vi "RT Driver VI.vi"(7 "Operation":T1, 11 "Device Reference in":T2 format="%.0x") -> (0 "Error Code":i32)   [LabVIEW 2019, in "Protection and Counter Addon Engine.lvlib"]
uses:
  Protection and Counter Addon Engine.lvlib
  <vilib>/NI VeriStand/Custom Device API/Custom Device Item Ref.ctl
  <vilib>/NI VeriStand/Custom Device API/Hardware Interface Driver VI Operation.ctl
  <vilib>/NI/NIVS Inline Async API/_VS Inline Async API/VS Inline Async API/VS Inline Async API.lvclass
  Types/RT Async Engine Settings.ctl
  SubModules/Frame-Protection-Support/Source/Engine/Types/RT Frame Settings.ctl
  SubModules/Frame-Protection-Support/Source/Shared/Types/Exported Frame Type.ctl
  SubModules/Frame-Protection-Support/Source/Engine/Types/RT Protection Configuration.ctl
  SubModules/Frame-Protection-Support/Source/Shared/Types/Protection Type.ctl
  SubModules/Frame-Protection-Support/Source/Shared/Types/XNET Signal Configuration.ctl
  SubModules/Frame-Protection-Support/Source/Shared/Types/Exported Counter Settings.ctl
  SubModules/Frame-Protection-Support/Source/Shared/Types/Exported Event Trigger Type.ctl
  Addon Shared/Types/XNET Settings.ctl
  SubModules/Frame-Protection-Support/Source/Shared/Types/RT_Incoming_Signal_Info.ctl
  SubModules/Frame-Protection-Support/Source/Shared/Types/RT Exported Signal Settings.ctl
  Addon Shared/Types/Exported.OnCompile.ctl
  SubModules/Frame-Protection-Support/Source/Shared/Types/Exported Frame Settings.ctl
  SubModules/Frame-Protection-Support/Source/Shared/Types/Exported Protection Settings.ctl
  Addon Shared/Types/986x.ctl
  SubModules/Frame-Protection-Support/Source/Shared/Types/Incoming Signal Info.ctl
  SubModules/Frame-Protection-Support/Source/Shared/Types/Exported Signal Settings.ctl
  <vilib>/NI/NIVS Inline Async API/_VS Inline Async API/VS Inline Async API/Types/Error Handling Settings.ctl
  <vilib>/NI/NIVS Inline Async API/_VS Inline Async API/VS Inline Async API/VS Inline Async API.lvclass/VS Inline Async API.ctl
  <vilib>/NI/NIVS Inline Async API/_Data Access Engine/Data Access Engine/Data Access Engine.lvclass/Data Access Engine.ctl
  <vilib>/NI/NIVS Inline Async API/_Data Access Engine/Access Type Classes/Write/Write.lvclass/Write.ctl
  <vilib>/NI/NIVS Inline Async API/_Data Access Engine/Access Type Classes/ReadWrite/ReadWrite.lvclass/ReadWrite.ctl
  <vilib>/NI/NIVS Inline Async API/_Data Access Engine/Access Type Classes/Read/Read.lvclass/Read.ctl
  <vilib>/NI/NIVS Inline Async API/_Data Access Engine/Data Access Engine/Methods/Data.Engine.Read Data from HW.vi
  <vilib>/NI/NIVS Inline Async API/_VS Inline Async API/Error Handling Process/SubVIs/Error.GetError.vi
  <vilib>/NI/NIVS Inline Async API/_Data Access Engine/Data Access Engine/Methods/Data.Engine.Write Data to HW.vi
  <vilib>/NI/NIVS Inline Async API/_Data Access Engine/Access Type Classes/ReadWrite/ReadWrite.EngineData.vi
  <vilib>/NI/NIVS Inline Async API/_Data Access Engine/Access Type Classes/Write/Write.EngineData.vi
  <vilib>/NI/NIVS Inline Async API/_Data Access Engine/Access Type Classes/Read/Read.EngineData.vi
  <vilib>/NI VeriStand/Custom Device API/NI VeriStand - Get Channel Value by Data Reference.vi
  <vilib>/NI VeriStand/Custom Device API/NI VeriStand - Set Channel Value by Data Reference.vi
  <vilib>/NI VeriStand/Custom Device API/NI VeriStand - Get Channel Values by Block Data Reference.vi
  Addon Shared/SubVIs/GUID Lookup.vi
  <vilib>/NI VeriStand/Custom Device API/Get Item Property (Variant).vi
  <vilib>/Utility/SystemLogging/Write to System Log.vi
  <vilib>/NI VeriStand/Custom Device API/Global Data Refs.vi
  <vilib>/NI VeriStand/Custom Device API/Custom Device API.lvlib
  Addon Shared/Protection and Counter Addon Shared.lvlib
  SubModules/Frame-Protection-Support/Source/Shared/Protection and Counter Support Shared.lvlib
  <vilib>/NI VeriStand/Custom Device Tools/Custom Device Utility Library/Custom Device Utility Library.lvlib
  SubModules/Frame-Protection-Support/Source/Engine/Protection and Counter Support Engine.lvlib
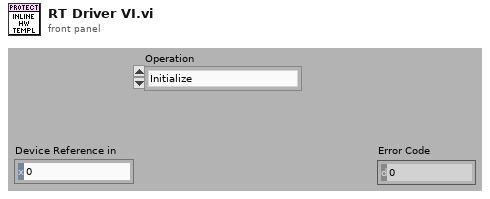
[diagram p1: front panel]
types:
  T1 = typedef "Custom Device API.lvlib/Hardware Interface Driver VI Operation.ctl" = enum16{"Initialize", "Start", "Read Data from HW", "Write Data to HW", "Close"}
  T2 = typedef "Custom Device API.lvlib/Custom Device Item Ref.ctl" = u64
  T3 = typedef "Protection and Counter Addon Engine.lvlib/RT Async Engine Settings.ctl" = cluster{"Name":string, "Priority":i32, "CAN Session":refnum<k21>, "Frame Count":i32, "Frames":T4[], "FPGA Session":u32, "XNET Settings":T11, "Incoming Frame Session":refnum<k21>, "Incoming Session Invalid":bool, "Incoming Signal Info":T12, "Signal Values":dbl[]}
  T4 = typedef "Protection and Counter Support Engine.lvlib/RT Frame Settings.ctl" = cluster{"Type":T5, "Frame ID":u32, "Payload Length":u32, "VS Offset":i32, "VS Length":i32, "Frame Conversion":refnum<k21>, "Frame.Data":dbl[], "Generation Period":u32, "Time Since Last Generation":u32, "Generation Iterations":u32, "Generation Counter":u32, "Has Protection?":bool, "Protection Configurations":T6[], "Has Counter?":bool, "Counter Configurations":T9[], "Has Disable?":bool, "Disable VS Index":i32, "Transmit Trigger":T10, "Trigger VS Index":i32}
  T5 = typedef "Protection and Counter Support Shared.lvlib/Exported Frame Type.ctl" = enum16{"Periodic", "Event", "Periodic/Event"}
  T6 = typedef "Protection and Counter Support Engine.lvlib/RT Protection Configuration.ctl" = cluster{"Protection Frame Index":i32, "Protection Type":T7, "Data Indeces":i32[], "Data Array":dbl[], "Check Sum Conversion":refnum<k21>, "CRC Channels":T8[], "Protection VS Index":i32, "Counter Data Index":i32, "Override Index":i32, "Override Value Index":i32}
  T7 = typedef "Protection and Counter Support Shared.lvlib/Protection Type.ctl" = enum16{"Arb ID + Bytes Checksum with Inversion", "Arb ID + Bytes CRC with Inversion", "Reversed Raw Signal Checksum with Inversion", "Concatenated Two's Compliment"}
  T8 = typedef "Protection and Counter Support Shared.lvlib/XNET Signal Configuration.ctl" = cluster{"Start Bit":i32, "Name":string, "Number of bits":i32, "Scale":dbl, "Offset":dbl, "Data Type":u32, "Counter":bool}
  T9 = typedef "Protection and Counter Support Shared.lvlib/Exported Counter Settings.ctl" = cluster{"Frame Index":i32, "Max Count":dbl, "VS Index":i32, "Bit Length":i64, "Override Index":i32, "Override Value Index":i32}
  T10 = typedef "Protection and Counter Support Shared.lvlib/Exported Event Trigger Type.ctl" = enum16{"Channel value change", "Trigger channel (not zero)", "Channel value change or trigger channel (not zero)", "Trigger channel (any value change)", "Channel value change or trigger channel (any value change)"}
  T11 = typedef "Protection and Counter Addon Shared.lvlib/XNET Settings.ctl" = cluster{"Database":refnum<k21>, "Cluster":refnum<k21>, "Port":string, "Baud rate [Bd]":u64, "Termination":u32, "CAN I/O Mode":u32, "FD Baud rate [Bd]":u64, "Priority":i32, "Use Legacy":bool, "FD ISO Mode":u32}
  T12 = typedef "RT_Incoming_Signal_Info.ctl" = cluster{"Signal_Valid_Values":dbl[], "Signal Names":string[], "Signal Settings Out":T13[], "Frame Receive Time Values":timestamp[], "ProtCtr Sig Values":dbl[], "All Sig Values":dbl[]}
  T13 = typedef "RT Exported Signal Settings.ctl" = cluster{"Is Protection":bool, "Is Counter":bool, "Signal Name":string, "Counter Configuration":T9, "Valid_Sig_Ref_Index":i32, "Frame ID":u32, "Payload Length":u32, "Protection Configuration":T6, "Frame Index":i32, "All Signal Index":i32}
  T14 = cluster{"Process":refnum<class "VS Inline Async API.lvclass">, "RT Configuration":T3}
  T15 = typedef "VS Inline Async API.lvlib/VS Inline Async API.lvclass/Error Handling Settings.ctl" = cluster{"Write to SystemLog (F)":bool}
  T16 = typedef "Protection and Counter Addon Shared.lvlib/Exported.OnCompile.ctl" = cluster{"Name":string, "XNET Settings":T11, "Frames":T17[], "986x Support":T19, "Incoming Signal Info":T20, "Incoming Frames":T17[]}
  T17 = typedef "Protection and Counter Support Shared.lvlib/Exported Frame Settings.ctl" = cluster{"Type":T5, "Frame ID":u32, "Payload Length":u32, "Signal XNET Paths":string[], "Frame.PrevData":dbl[], "VS Offset":i32, "VS Length":i32, "Generation Period":u32, "Has Protection?":bool, "Protection Configurations":T18[], "Has Counter":bool, "Counter Configurations":T9[], "Has Disable?":bool, "Disable VS Index":i32, "Transmit Trigger":T10, "Trigger VS Index":i32}
  T18 = typedef "Protection and Counter Support Shared.lvlib/Exported Protection Settings.ctl" = cluster{"Protection Frame Index":i32, "Protection Type":T7, "Data Indeces":i32[], "Initialized Data Array":dbl[], "Protection Signal XNET Paths":string[], "CRC Channels":T8[], "Protection VS Update Index":i32, "Override Index":i32, "Override Value Index":i32}
  T19 = typedef "Protection and Counter Addon Shared.lvlib/986x.ctl" = cluster{"Enable":bool, "RIO Device":string, "Bitfile":path}
  T20 = typedef "Incoming Signal Info.ctl" = cluster{"Signal Settings Out":T21[], "Signal_Valid_Values":dbl[], "Signal Names":string[], "ProtCtrValues":dbl[], "AllSigValues":dbl[]}
  T21 = typedef "Exported Signal Settings.ctl" = cluster{"Is Protection":bool, "Is Counter":bool, "Signal Name":string, "Counter Configuration":T9, "Protection Configuration":T18, "Valid_Sig_Ref_Index":i32, "Frame ID":u32, "Payload Length":u32, "Frame Index":i32, "All Signal Index":i32}
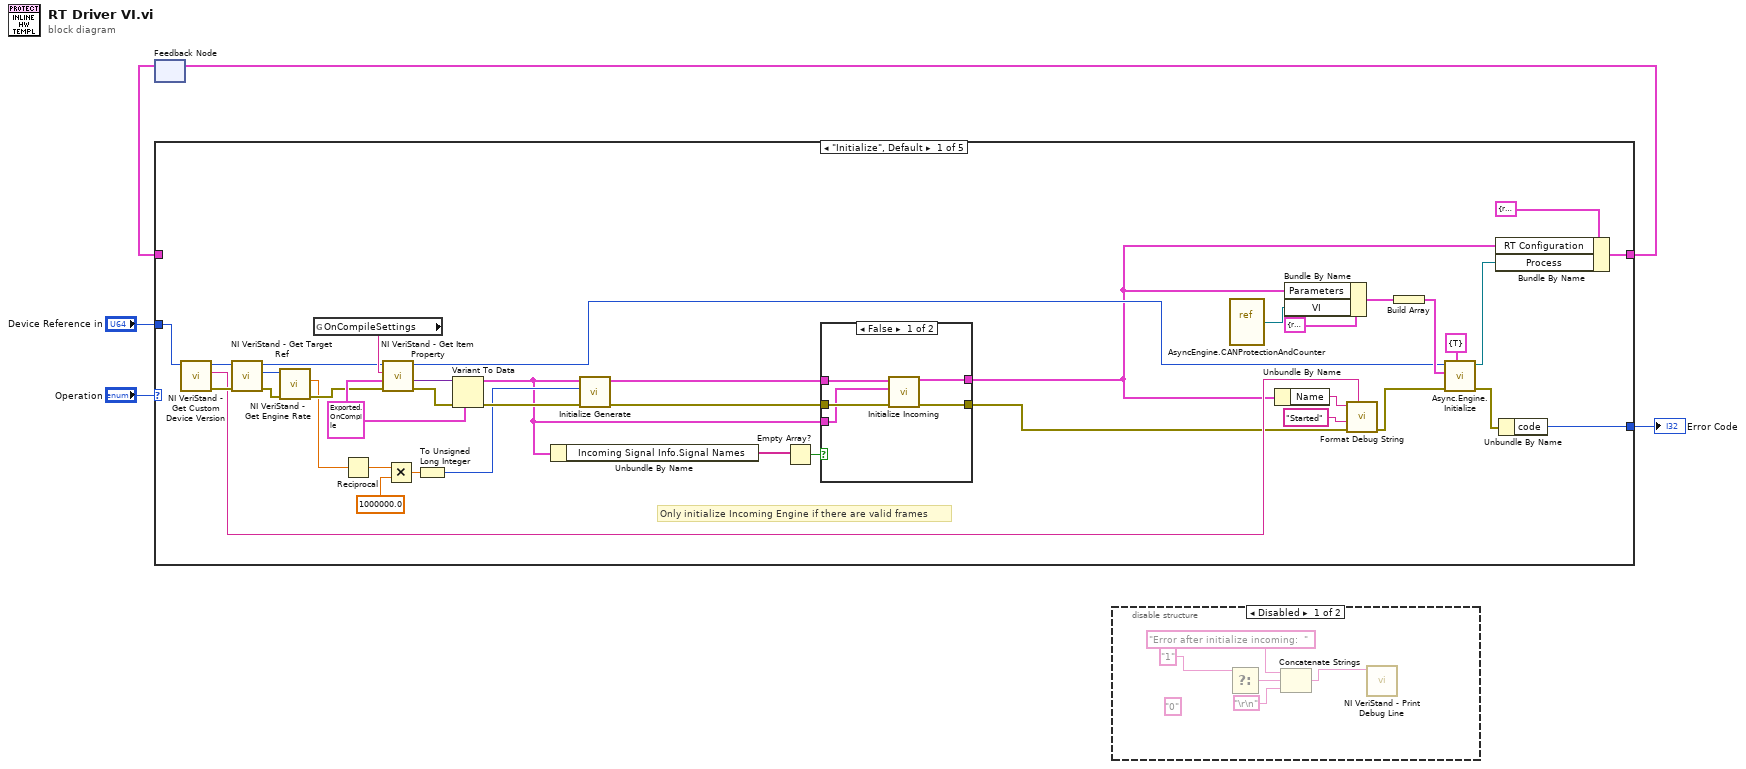
[diagram p0: block diagram]
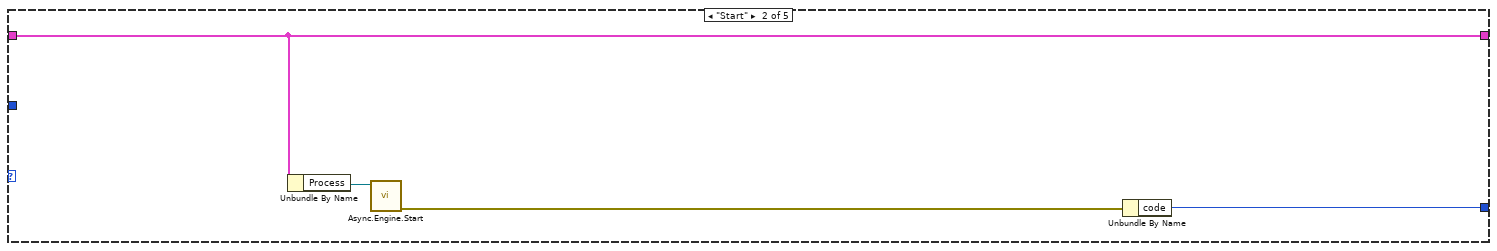
[diagram p4: hidden frame]
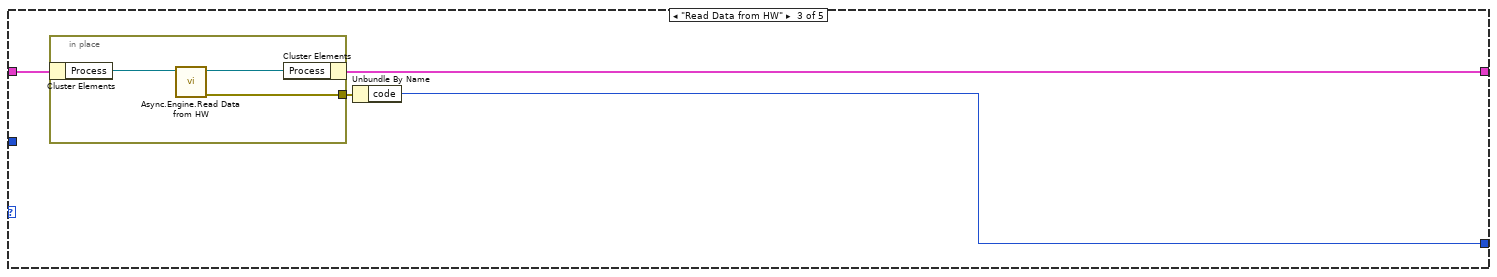
[diagram p5: hidden frame]
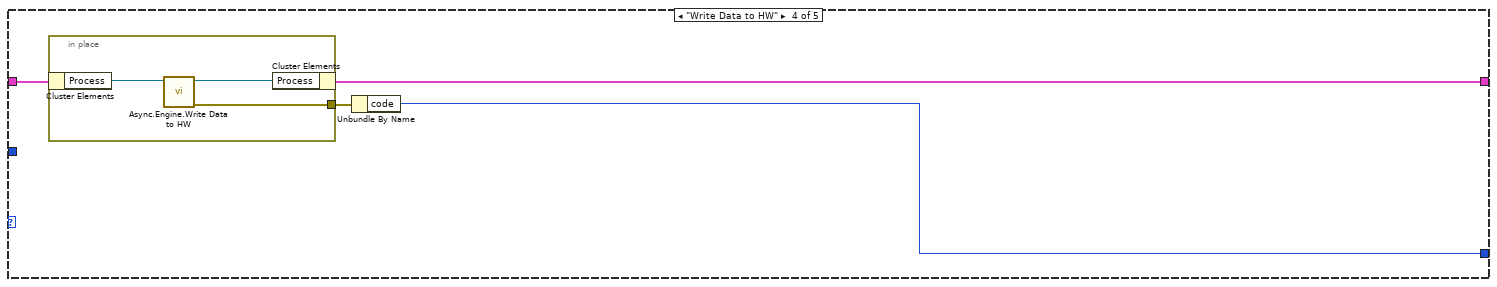
[diagram p6: hidden frame]
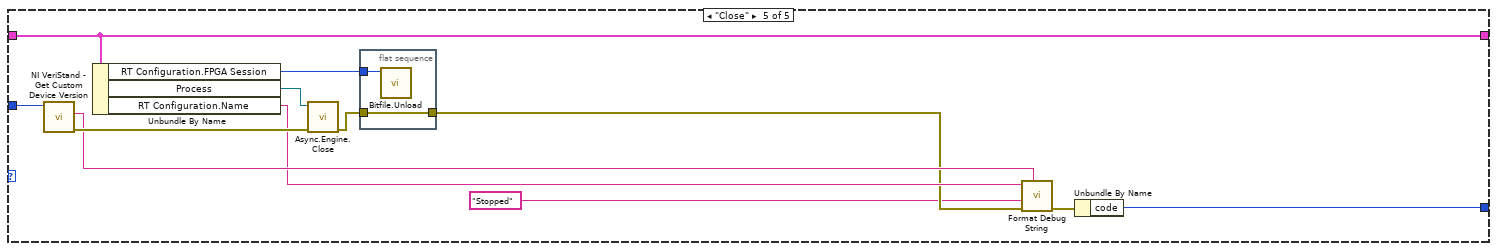
[diagram p7: hidden frame]
diagram:
  n1 = feedback #1() -> (w3:T14)  [unwired: 1 out]
  n2 = case shown="\"Initialize\", Default" "Operation" {
    tunnel: [w43 w52 w58 w66 w78] -> w4
    tunnel: w3 -> [_ w52 w59 w65 w78]
    tunnel: [w44 w55 w56 w63 w73] -> w2
    tunnel: "Device Reference in" -> [w42 _ _ _ w81]
    frame "Initialize", Default {
      w32 = T16 {"Name"="", "XNET Settings"={"Database"="", "Cluster"="", "Port"="", "Baud rate [Bd]"=500000, "Termination"=1, "CAN I/O Mode"=0, "FD Baud rate [Bd]"=500000, "Priority"=100, "Use Legacy"=FALSE, "FD ISO Mode"=0}, "Frames"=[], "986x Support"={"Enable"=FALSE, "RIO Device"="", "Bitfile"=path ""}, "Incoming Signal Info"={"Signal Settings Out"=[], "Signal_Valid_Values"=[], "Signal Names"=[], "ProtCtrValues"=[], "AllSigValues"=[]}, "Incoming Frames"=[]} ("Cluster")
      # "Only initialize Incoming Engine if there are valid frames"
      n3 = call <vilib>:"NI VeriStand - Get Custom Device Version.vi"("Device Ref in"=w42) -> ("error out"=w26:errorcluster, "Value"=w15:string, "Device Ref out"=w35:T2)  [unwired: 8 in]
      n4 = call <vilib>:"NI VeriStand - Get Target Ref.vi"("error in"=w26, "Item Ref in"=w35) -> ("error out"=w25:errorcluster, "Target Ref"=w27:T2, "Item Ref out"=w28:T2)  [unwired: 6 in, 1 out]
      n5 = call <vilib>:"NI VeriStand - Get Engine Rate.vi"("error in (no error)"=w25, "Item Ref in"=w27) -> ("error out"=w24:errorcluster, "Rate (Hz)"=w23:dbl)  [unwired: 7 in, 1 out]
      n6 = global read "GUID Lookup.vi" "OnCompileSettings"() -> (w36:string)
      n7 = Reciprocal(x=w23) -> (1/x=w22:dbl)
      n8 = call-poly <vilib>:"NI VeriStand - Get Item Property.vi"("error in (no error)"=w24, "Default Value"=w32, "Property Name"=w36, "Item Ref in"=w28) -> ("error out"=w33:errorcluster, "Value"=w34:variant, "Item Ref out"=w31:T2)  [unwired: 4 in, 1 out]
      n9 = Multiply(x=w22, y=1000000.0) -> (x*y=w20:dbl)
      n10 = To Unsigned Long Integer(number=w20) -> (unsigned 32bit integer=w19:u32)
      n11 = Variant To Data(error in=w33, type=w32, Variant=w34) -> (data=w12:T16, error out=w30:errorcluster)
      n12 = Unbundle By Name(w12) -> ("Incoming Signal Info.Signal Names"=w14:string[])
      n13 = call "Initialize Generate.vi"("error in (no error)"=w30, "PCL (usec)"=w19, "OnCompile Variables"=w12) -> ("error out"=w8:errorcluster, "RT Configuration"=w9:T3)  [unwired: 7 in]
      n14 = Empty Array?(array=w14) -> (empty?=w13:bool)
      n15 = case shown="False" w13 {
        tunnel: [w48 w51] -> w7
        tunnel: w8 -> [w49 w51]
        tunnel: w12 -> [w47 _]
        tunnel: w9 -> [w46 w50]
        tunnel: [w45 w50] -> w6
        frame False {
          n16 = call "Initialize Incoming.vi"("error in (no error)"=w49, "OnCompile Variables"=w47, "RT Configuration In"=w46) -> ("error out"=w48:errorcluster, "RT Configuration Out"=w45:T3)  [unwired: 7 in]
        }
        frame True {
        }
      }
      n17 = vi-ref "AsyncEngine.CANProtectionAndCounter.vi"() -> (w29:refnum<vi>)
      n18 = Unbundle By Name(w6) -> ("Name"=w17:string)
      n19 = Bundle By Name(cluster=cluster{"VI":refnum<vi>, "Parameters":variant} {"VI"=refnum, "Parameters"=variant} ("Process"), "Parameters"=w6, "VI"=w29) -> (w39:cluster{"VI":refnum<vi>, "Parameters":variant})
      n20 = call "Format Debug String.vi"("Version"=w15, "error in (no error)"=w7, "State"="Started", "Name"=w17) -> ("error out"=w10:errorcluster)  [unwired: 7 in]
      n21 = Build Array(w39) -> (w38:cluster{"VI":refnum<vi>, "Parameters":variant}[])
      n22 = call <vilib>:"Async.Engine.Initialize.vi"("Error Log Settings"=T15 {"Write to SystemLog (F)"=TRUE}, "error in (no error)"=w10, "Processes"=w38, "Custom Device Ref"=w31) -> ("error out"=w11:errorcluster, "Async"=w41:refnum<class "VS Inline Async API.lvclass">)  [unwired: 6 in]
      n23 = Bundle By Name(cluster=T14 {"Process"=refnum, "RT Configuration"={"Name"="", "Priority"=100, "CAN Session"="", "Frame Count"=0, "Frames"=[], "FPGA Session"=0, "XNET Settings"={"Database"="", "Cluster"="", "Port"="", "Baud rate [Bd]"=0, "Termination"=0, "CAN I/O Mode"=0, "FD Baud rate [Bd]"=500000, "Priority"=100, "Use Legacy"=FALSE, "FD ISO Mode"=0}, "Incoming Frame Session"="", "Incoming Session Invalid"=FALSE, "Incoming Signal Info"={"Signal_Valid_Values"=[], "Signal Names"=[], "Signal Settings Out"=[], "Frame Receive Time Values"=[], "ProtCtr Sig Values"=[], "All Sig Values"=[]}, "Signal Values"=[]}} ("input cluster"), "RT Configuration"=w6, "Process"=w41) -> (w43:T14)
      n24 = Unbundle By Name(w11) -> ("code"=w44:i32)
    }
    frame "Start" {
      n25 = Unbundle By Name(w52) -> ("Process"=w54:refnum<class "VS Inline Async API.lvclass">)
      n26 = call <vilib>:"Async.Engine.Start.vi"("VS Inline Async API in"=w54) -> ("error out"=w53:errorcluster)  [unwired: 9 in, 1 out]
      n27 = Unbundle By Name(w53) -> ("code"=w55:i32)
    }
    frame "Read Data from HW" {
      n28 = in-place {
        in-place-border: [w60] -> w57
        n29 = in-place-cluster #2(w59) -> ("Process"=w62:refnum<class "VS Inline Async API.lvclass">)
        n30 = call <vilib>:"Async.Engine.Read Data from HW.vi"("Async in"=w62) -> ("error out"=w60:errorcluster, "Async out"=w61:refnum<class "VS Inline Async API.lvclass">)  [unwired: 9 in]
        n31 = in-place-cluster #2("Process"=w61) -> (w58:T14)
      }
      n32 = Unbundle By Name(w57) -> ("code"=w56:i32)
    }
    frame "Write Data to HW" {
      n33 = in-place {
        in-place-border: [w67] -> w64
        n34 = in-place-cluster #3(w65) -> ("Process"=w69:refnum<class "VS Inline Async API.lvclass">)
        n35 = call <vilib>:"Async.Engine.Write Data to HW.vi"("VS Inline Async API in"=w69) -> ("error out"=w67:errorcluster, "VS Inline Async API out"=w68:refnum<class "VS Inline Async API.lvclass">)  [unwired: 9 in]
        n36 = in-place-cluster #3("Process"=w68) -> (w66:T14)
      }
      n37 = Unbundle By Name(w64) -> ("code"=w63:i32)
    }
    frame "Close" {
      n38 = call <vilib>:"NI VeriStand - Get Custom Device Version.vi"("Device Ref in"=w81) -> ("error out"=w77:errorcluster, "Value"=w76:string)  [unwired: 8 in, 1 out]
      n39 = Unbundle By Name(w78) -> ("RT Configuration.FPGA Session"=w79:u32, "Process"=w80:refnum<class "VS Inline Async API.lvclass">, "RT Configuration.Name"=w75:string)
      n40 = call <vilib>:"Async.Engine.Close.vi"("error in (no error)"=w77, "Async in"=w80) -> ("error out"=w70:errorcluster)  [unwired: 8 in, 1 out]
      n41 = flat-sequence {
        tunnel: w79 -> [w83]
        tunnel: w70 -> [w82]
        tunnel: [w82] -> w74
        frame #0 {
          n42 = call "Bitfile.Unload.vi"("Session"=w83) -> ()  [unwired: 11 in]
        }
      }
      n43 = call "Format Debug String.vi"("Version"=w76, "error in (no error)"=w74, "State"="Stopped", "Name"=w75) -> ("error out"=w71:errorcluster)  [unwired: 7 in]
      n44 = Unbundle By Name(w71) -> ("code"=w73:i32)
    }
  }
  "Error Code" <- w2
  n45 = feedback-in #1(w4) -> ()
  n46 = disable-structure shown="Disabled" {
    frame Disabled {
      (unwired) "0" ("string")
      n47 = Select(t="1" ("string")) -> (s? t:f=w84:string)  [unwired: 2 in]
      n48 = Concatenate Strings("Error after initialize incoming:  " ("string"), w84, "\r\n") -> (w86:string)
      n49 = call <vilib>:"NI VeriStand - Print Debug Line.vi"("Message"=w86) -> ()  [unwired: 10 in, 1 out]
    }
    frame Enabled {
    }
  }
